vi "InitCurrentPressure.vi"   [LabVIEW 2013]
uses:
  GlobalVariables/CurrentPressure.vi
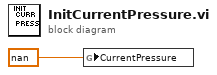
[diagram p0: block diagram]
diagram:
  n1 = global write "CurrentPressure.vi" "CurrentPressure"(nan) -> ()
